vi "Read and Analyze Ringdowns.vi"() -> ()   [LabVIEW 2012]
uses:
  Reusable/General/Math Utilities.lvlib
  CRDS Class/Main Class/Controls/Get Tau Method.ctl
  <vilib>/measure/NI_MAPro.lvlib
  <vilib>/measure/maspectr.llb/FFT Power Spectral Density for 1 Chan.vi
  <vilib>/Analysis/4window.llb/windowTd.ctl
  <vilib>/Analysis/NI_AALPro.lvlib
  <vilib>/Analysis/NI_AALBase.lvlib
  <vilib>/Analysis/baseanly.llb/Mean (DBL).vi
panel:
  out "System Waveform Graph 2":dbl[](graph)
  in  "Ring 2":u16(ring) items=["Cell 1", "Cell 2", "Cell 3", "Cell 4", "Cell 5", "Cell 6", "Cell 7", "Cell 8"]
  out "tauOut 2":cluster{timestamp[], dbl[]}[](graph)
  out "Points Processed":i32
  in  "numSecs":i32=1
  in  "Ring":u16(ring) items=["Cell 1", "Cell 2", "Cell 3", "Cell 4", "Cell 5", "Cell 6", "Cell 7", "Cell 8"]
  in  "close":bool
  out "System Waveform Graph":i16[](graph)
  in  "plot":bool
  in  "read":bool
  out "Read Path":path
  out "tauOut":cluster{timestamp[], dbl[]}[](graph)
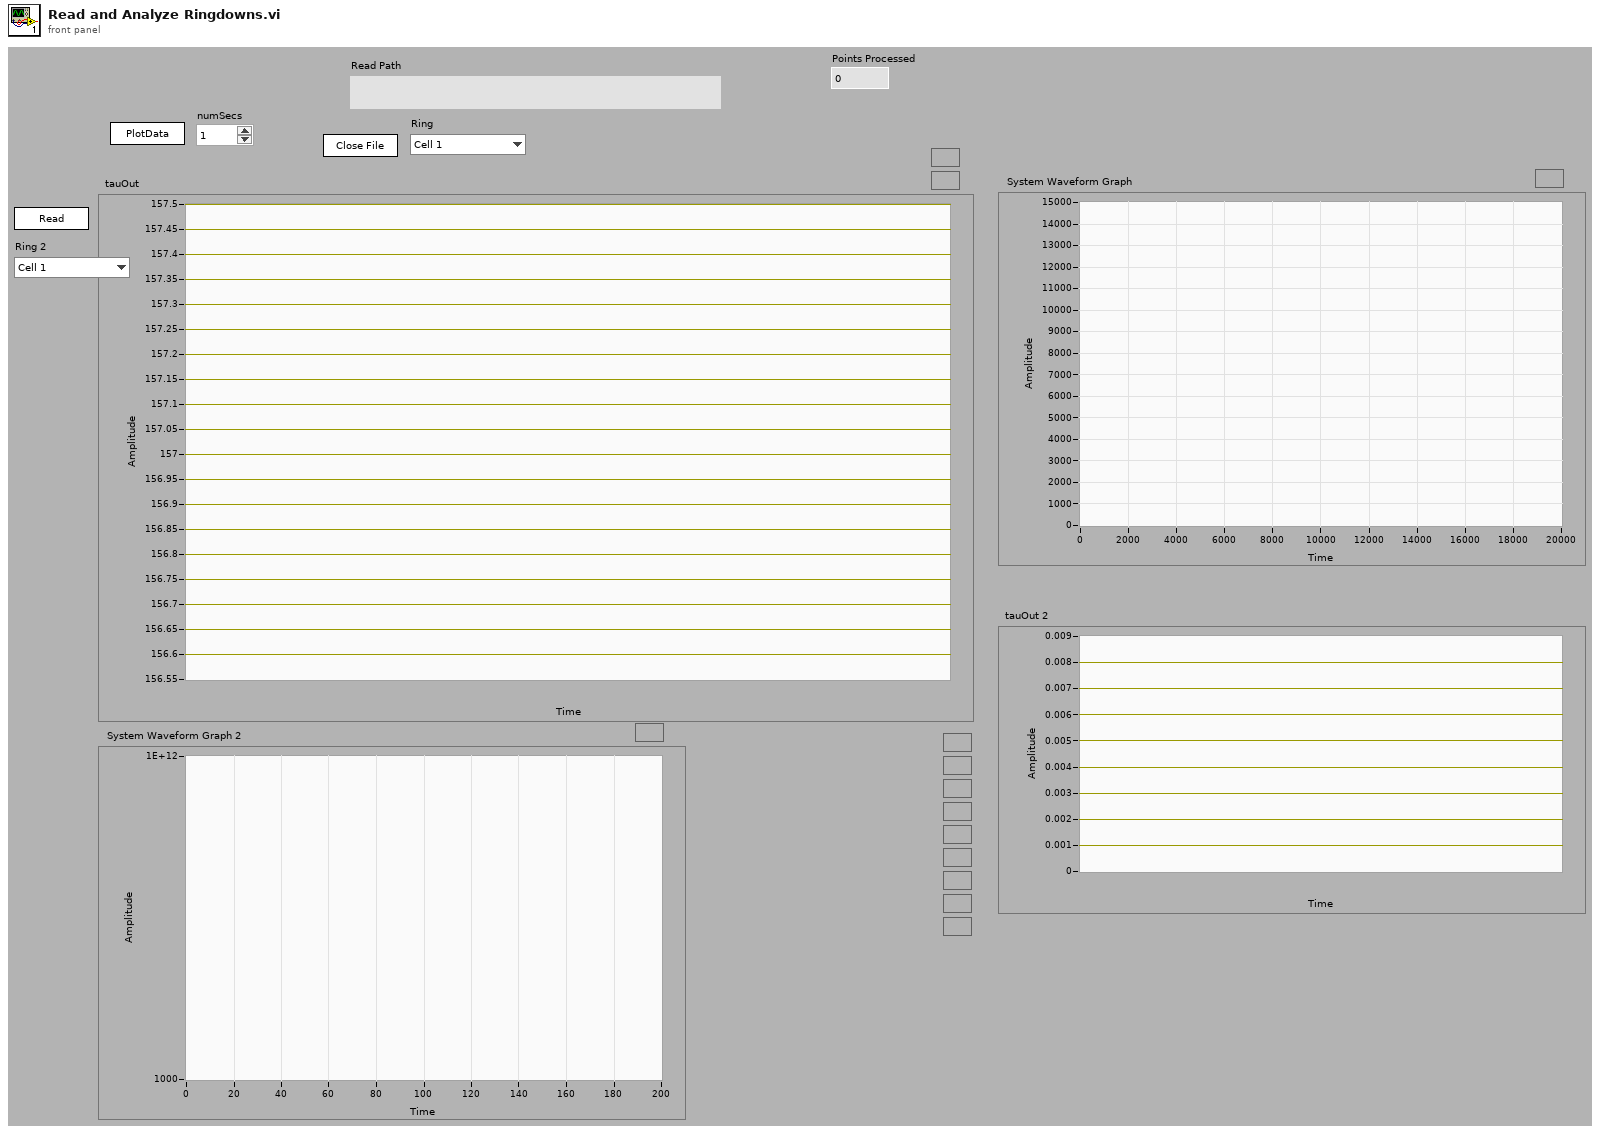
[diagram p1: front panel]
types:
  T1 = typedef "Get Tau Method.ctl" = enum8{"DFT-1", "DFT-5", "LRS"}
  T2 = typedef "NI_AALPro.lvlib/windowTd.ctl" = u32
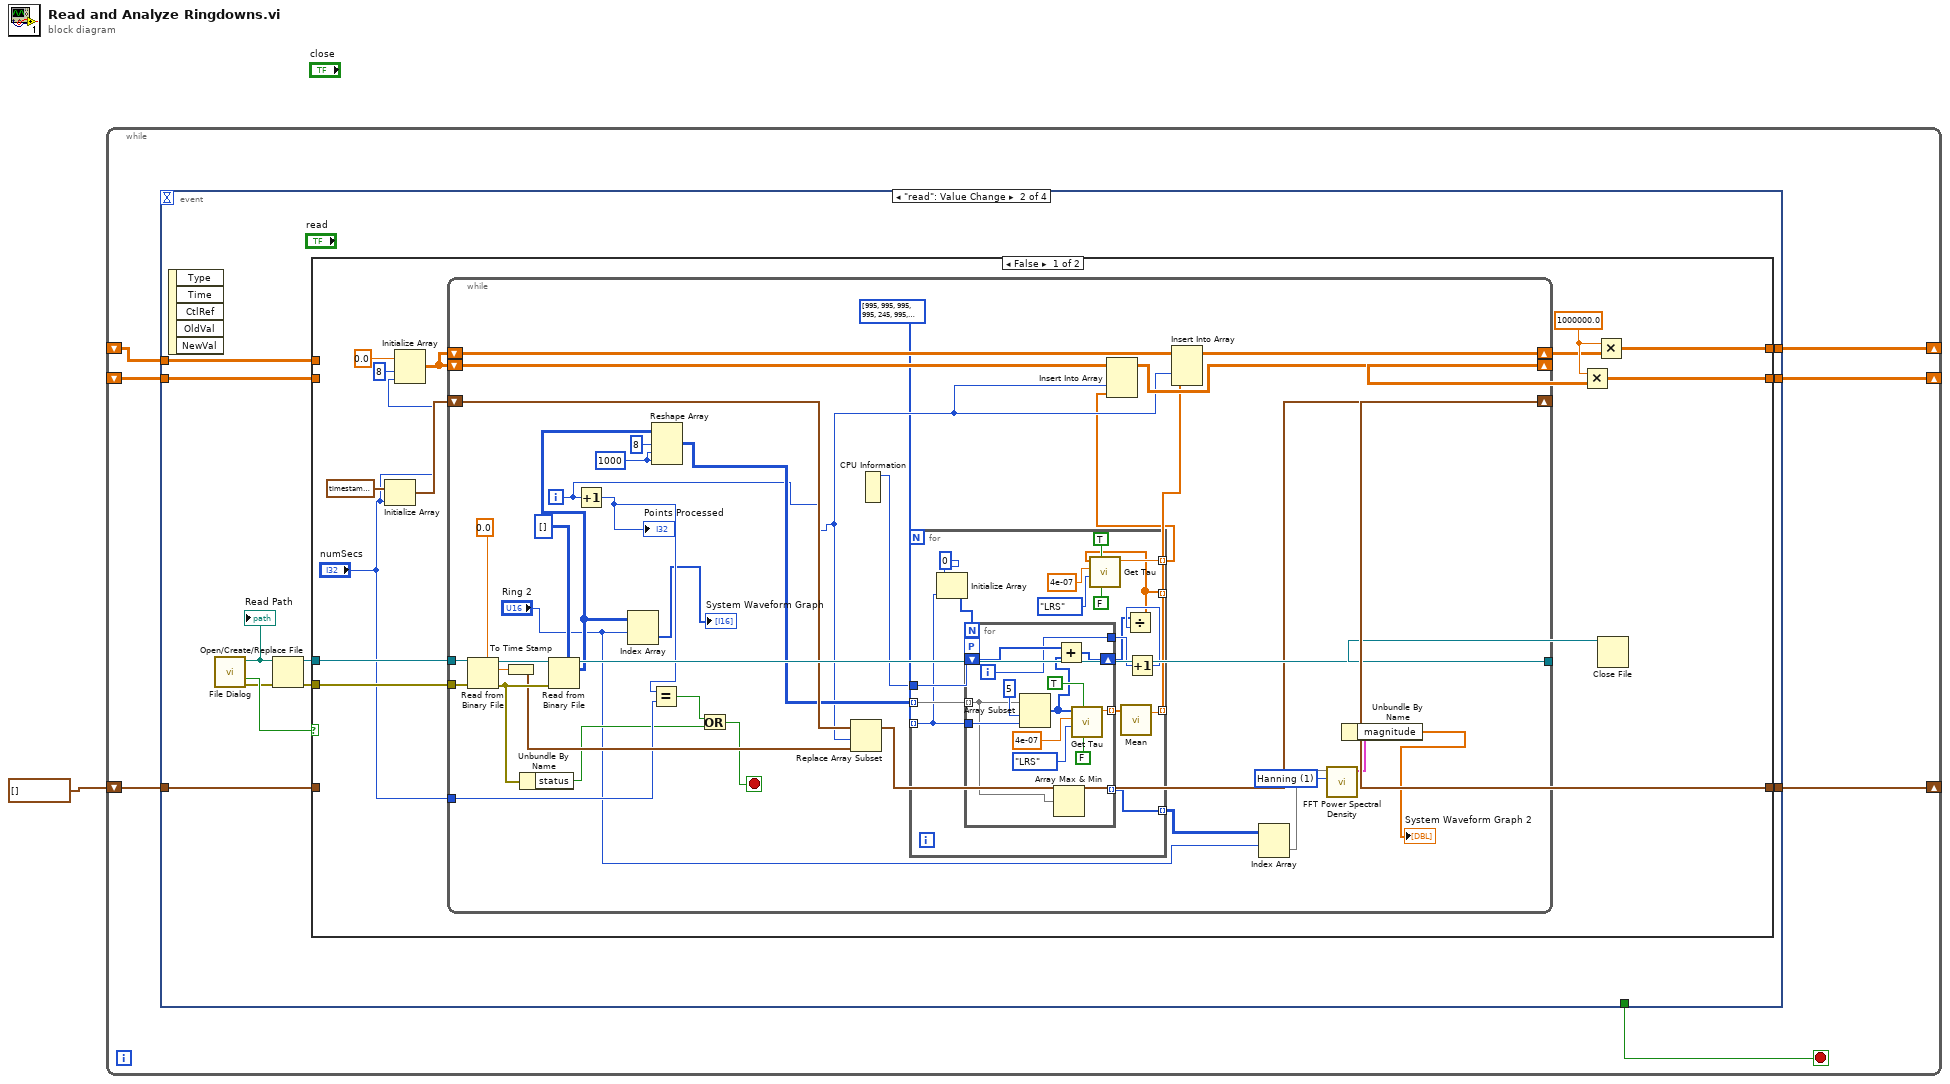
[diagram p0: block diagram]
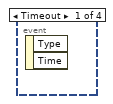
[diagram p2: hidden frame]
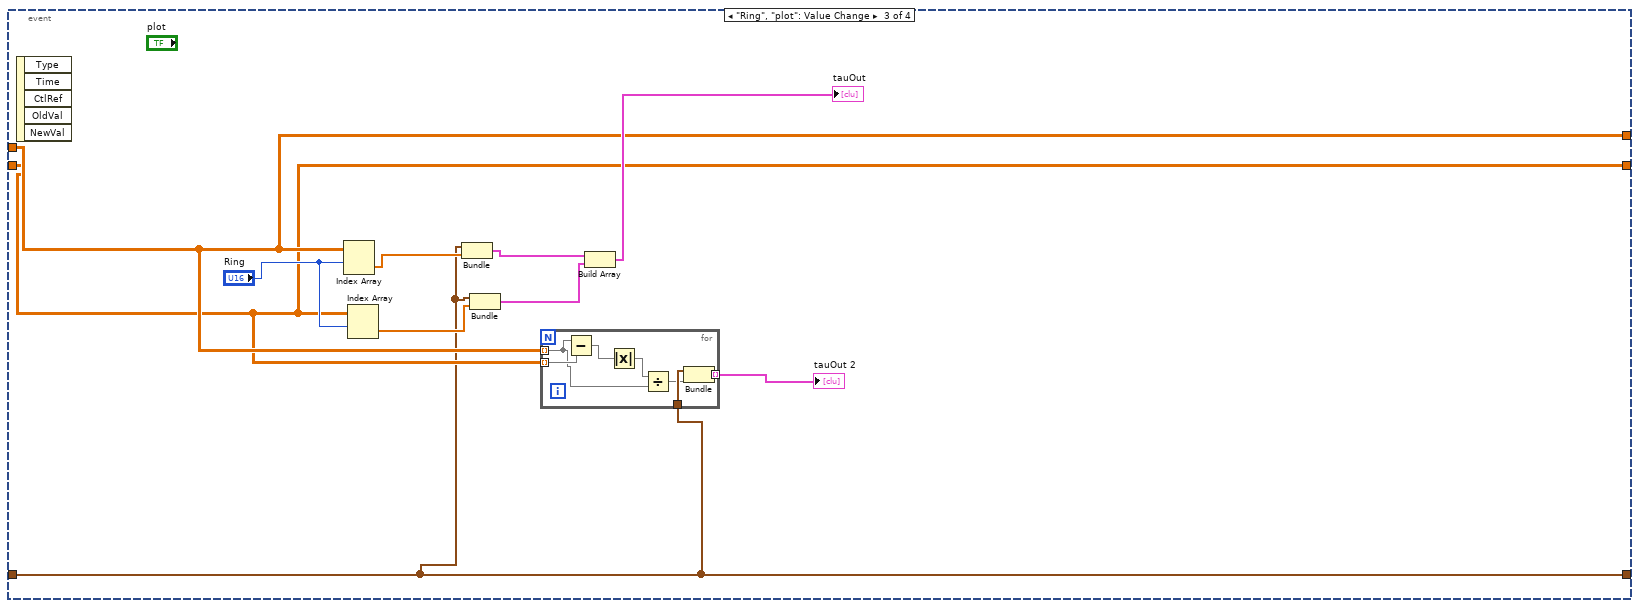
[diagram p4: hidden frame]
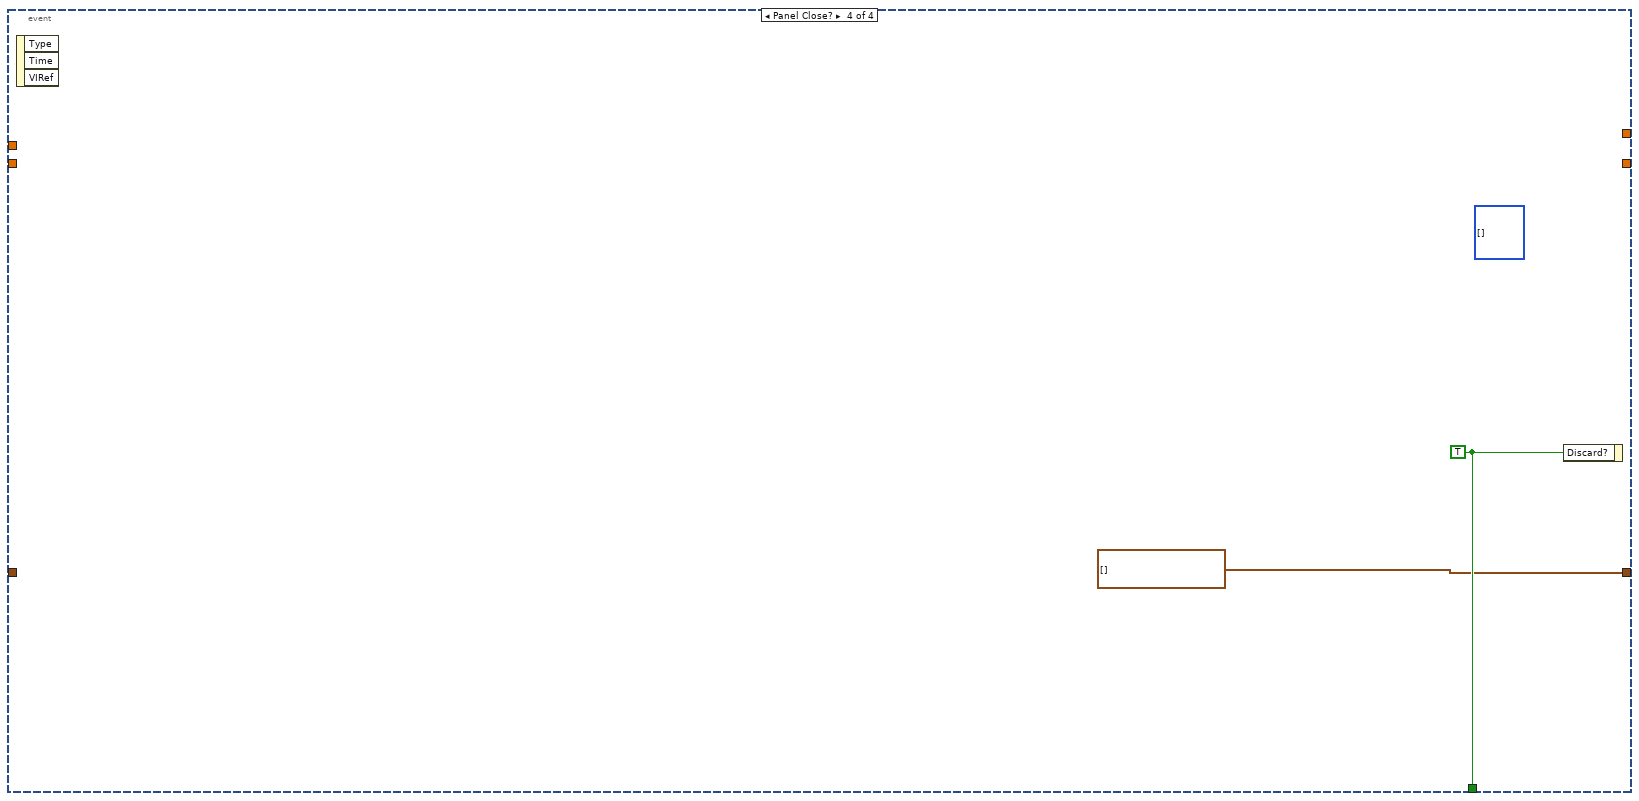
[diagram p5: hidden frame]
diagram:
  n1 = while {
    shift-right: [w7] -> _
    shift-left: timestamp[] [] -> [w8]
    shift-right: [w5] -> _
    shift-left: _ -> [w2]
    shift-right: [w4] -> _
    shift-left: _ -> [w3]
    stop <- w6 stop-if-true
    n2 = event shown="[1] \"read\": Value Change" {
      selector: _ -> [_ _ _ _]
      dyn-events: _ -> [_ _ _ _]
      timeout: _ -> [_ _ _ _]
      tunnel: w8 -> [_ w16 w105 _]
      tunnel: [_ w15 w105 timestamp[] []] -> w7
      tunnel: [_ _ _ w122] -> w6
      tunnel: [_ w14 w106 _] -> w5
      tunnel: [_ w13 w107 _] -> w4
      tunnel: w3 -> [_ w12 w107 _]
      tunnel: w2 -> [_ w11 w106 _]
      event Timeout {
        n3 = event-data() -> ()  [unwired: 1 in, 2 out]
      }
      event "read": Value Change {
        n4 = event-data() -> ()  [unwired: 1 in, 5 out]
        n5 = call "File Dialog"() -> ("selected path"=w10:path, "cancelled"=w19:bool, "error out"=w9:errorcluster)  [unwired: 12 in, 1 out]
        "Read Path" <- w10
        n6 = Open/Create/Replace File(file path (use dialog)=w10, error in=w9) -> (refnum out=w17:refnum<file>, error out=w18:errorcluster)  [unwired: 4 in, 1 out]
        n7 = case shown="False" w19 {
          tunnel: w18 -> [w33 _]
          tunnel: w17 -> [w34 _]
          tunnel: w16 -> [_ w103]
          tunnel: [w30 w103] -> w15
          tunnel: [w22 w101] -> w14
          tunnel: [w21 w102] -> w13
          tunnel: w12 -> [_ w102]
          tunnel: w11 -> [_ w101]
          frame False {
            w24 = 1000000.0
            n8 = Initialize Array(timestamp(0 s since 1904-01-01), "numSecs") -> (w31:timestamp[])
            n9 = Initialize Array(0.0, 8 ("dimension size"), "numSecs") -> (w27:dbl[][])
            n10 = while {
              tunnel: w34 -> [w70]
              tunnel: w33 -> [w69]
              shift-right: [w61] -> w30
              shift-left: w31 -> [w62]
              tunnel: [w65] -> w20
              shift-right: [w58] -> w25
              shift-left: w27 -> [w59]
              shift-right: [w56] -> w23
              shift-left: w27 -> [w57]
              tunnel: "numSecs" -> [w53]
              i -> [w50]
              stop <- w43 stop-if-true
              w37 = T2 1 items=["Rectangle"=0, "Hanning"=1, "Hamming"=2, "Blackman-Harris"=3, "Exact Blackman"=4, "Blackman"=5, "Flat Top"=6, "4 Term B-Harris "=7, "7 Term B-Harris"=8, "Low Sidelobe"=9, "Blackman Nuttall"=11, "Triangle"=30, "Bartlett-Hanning"=31, "Bohman"=32, "Parzen"=33, "Welch"=34, "Kaiser"=60, "Dolph-Chebyshev"=61, "Gaussian"=62] ("window")
              w54 = 1000 ("dimension size")
              n11 = Read from Binary File(5:0.0, 8:w69, 11:w70) -> (0:w64:errorcluster, 2:w63:dbl, 3:w67:refnum<file>)  [unwired: 3 in, 1 out]
              n12 = To Time Stamp(1:w63) -> (0:w60:timestamp)
              n13 = Unbundle By Name(w64) -> ("status"=w44:bool)
              n14 = Read from Binary File(5:i16[][] [], 8:w64, 11:w67) -> (2:w42:i16[][], 3:w65:refnum<file>)  [unwired: 3 in, 2 out]
              n15 = Increment(x=w50) -> (x+1=w52:i32)
              "Points Processed" <- w52
              n16 = Index Array(array=w42, index (row)="Ring 2") -> (element=→"System Waveform Graph":i16[])  [unwired: 1 in]
              n17 = Equal?(x=w52, y=w53) -> (x = y?=w45:bool)
              n18 = Reshape Array(w42, i16 8 ("dimension size"), w54, w54) -> (w51:i16[][][])
              n19 = Or(x=w45, y=w44) -> (x .or. y?=w43:bool)
              n20 = Replace Array Subset(array=w62, new element=w60, index=w50) -> (w61:timestamp[])
              n21 = CPU Information() -> (4:w48:i32)  [unwired: 3 out]
              n22 = for {
                tunnel: i32[] [995, 995, 995, 995, 245, 995, 995, 245] -> [w77] mode=indexing
                tunnel: w48 -> [w87]
                tunnel: [w85] -> w47 mode=indexing
                tunnel: w51 -> [w86] mode=indexing
                tunnel: [w76] -> w46 mode=indexing
                tunnel: [w72] -> _ mode=indexing
                tunnel: [w71] -> w40 mode=indexing
                n23 = Initialize Array(0 ("index"), w77) -> (w82:i32[])
                n24 = for {
                  tunnel: w77 -> [w99]
                  tunnel: [w94] -> w84 mode=indexing
                  workers-P: w87 -> [_]
                  tunnel: w86 -> [w89] mode=indexing
                  shift-right: [w91] -> w73
                  shift-left: w82 -> [w92]
                  tunnel: [w90] -> w75
                  tunnel: [w88] -> w71 mode=indexing
                  i -> [w90]
                  n25 = Array Subset(array=w89, index=5, length=w99) -> (w93:i16[])
                  n26 = Array Max & Min(array=w89) -> (max value=w88:i16)  [unwired: 3 out]
                  n27 = Add(x=w92, y=w93) -> (x+y=w91:i32[])
                  n28 = call "Get Tau.vi"("ErrorCallOn"=FALSE, "init"=TRUE, "CalType"=Get_Tau_Method."LRS", "Dt"=4e-07, "X"=w93) -> ("tau"=w94:dbl)  [unwired: 3 in, 3 out]
                }
                n29 = call-poly <vilib>:"Mean.vi"("X"=w84) -> ("mean"=w85:dbl)  [unwired: 1 out]
                n30 = Increment(x=w75) -> (x+1=w74:i32)
                n31 = Divide(x=w73, y=w74) -> (x/y=w72:dbl[])
                n32 = call "Get Tau.vi"("ErrorCallOn"=FALSE, "init"=TRUE, "CalType"=Get_Tau_Method."LRS", "Dt"=4e-07, "X"=w72) -> ("tau"=w76:dbl)  [unwired: 3 in, 3 out]
              }
              n33 = Insert Into Array(array=w59, index (col)=w50, new element=w46) -> (w58:dbl[][])  [unwired: 1 in]
              n34 = Insert Into Array(array=w57, index (col)=w50, new element=w47) -> (w56:dbl[][])  [unwired: 1 in]
              n35 = Index Array(array=w40, index (row)="Ring 2") -> (element=w38:i16[])  [unwired: 1 in]
              n36 = call-poly <vilib>:"FFT Power Spectral Density.vi"("window"=w37, "time signal"=w38) -> ("power spectral density"=w36:cluster{"f0":dbl, "df":dbl, "magnitude":dbl[]})  [unwired: 6 in, 3 out]
              n37 = Unbundle By Name(w36) -> ("magnitude"=→"System Waveform Graph 2":dbl[])
            }
            n38 = Multiply(x=w24, y=w25) -> (x*y=w22:dbl[][])
            n39 = Multiply(x=w24, y=w23) -> (x*y=w21:dbl[][])
            n40 = Close File(refnum=w20) -> ()  [unwired: 1 in, 2 out]
          }
          frame True {
          }
        }
      }
      event "Ring", "plot": Value Change {
        n41 = event-data() -> ()  [unwired: 1 in, 5 out]
        n42 = Index Array(array=w107, index (row)="Ring") -> (element=w108:dbl[])  [unwired: 1 in]
        n43 = Index Array(array=w106, index (row)="Ring") -> (element=w109:dbl[])  [unwired: 1 in]
        n44 = Bundle(w105, w108) -> (w111:cluster{timestamp[], dbl[]})  [unwired: 1 in]
        n45 = Bundle(w105, w109) -> (w112:cluster{timestamp[], dbl[]})  [unwired: 1 in]
        n46 = for {
          tunnel: w107 -> [w117] mode=indexing
          tunnel: w106 -> [w118] mode=indexing
          tunnel: w105 -> [w116]
          tunnel: [w114] -> w104 mode=indexing
          n47 = Subtract(x=w117, y=w118) -> (x-y=w120:dbl[])
          n48 = Absolute Value(x=w120) -> (abs(x)=w119:dbl[])
          n49 = Divide(x=w119, y=w117) -> (x/y=w115:dbl[])
          n50 = Bundle(w116, w115) -> (w114:cluster{timestamp[], dbl[]})  [unwired: 1 in]
        }
        "tauOut 2" <- w104
        n51 = Build Array(w111, w112) -> (→"tauOut":cluster{timestamp[], dbl[]}[])
      }
      event Panel Close? {
        (unwired) i16[][][] []
        w122 = TRUE ("Discard?")
        n52 = event-data() -> ()  [unwired: 1 in, 3 out]
        n53 = event-data("Discard?"=w122) -> ()  [unwired: 1 in, 1 out]
      }
    }
  }
